vi "contains.vi"(0 "reference":refnum<class "PackageNode.lvclass">, 1 "point2D":T1 {"y" format="%.2f"; "x" format="%.2f"}, 2 "AdditionalMargin":i32, 5 "error in (no error)":errorcluster) -> (14 "reference out":refnum<class "PackageNode.lvclass">, 15 "contains":bool, 19 "error out":errorcluster)   [LabVIEW 2014, in "PackageNode.lvclass"]
doc: "contains"
uses:
  <resource>/Framework/Providers/Open_GDS/UML/PackageNode_class/PackageNode.lvclass
  <resource>/Framework/Providers/Open_GDS/UML/General/Point/Point Point2D.ctl
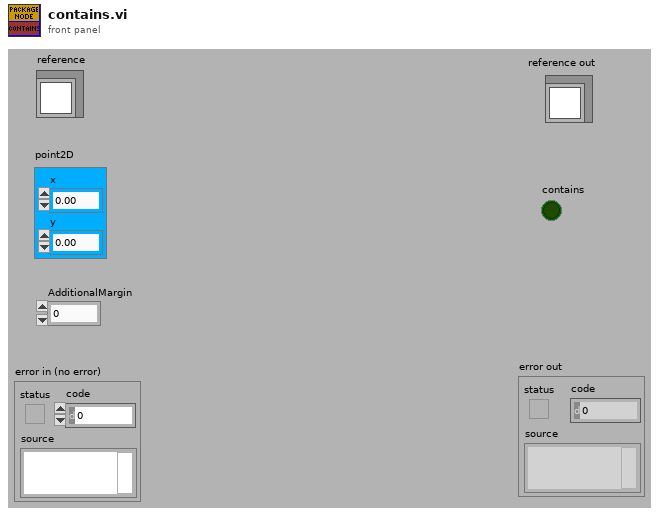
[diagram p1: front panel]
types:
  T1 = typedef "Point Point2D.ctl" = cluster{"x":dbl, "y":dbl}
  T2 = typedef "PackageNode.lvclass/ObjectAttributes.ctl" = cluster{"Base class":T3, "name":string, "contents":refnum<class "MultiLineString.lvclass">, "DEFAULT_TOP_WIDTH":i32, "DEFAULT_TOP_HEIGHT":i32, "DEFAULT_WIDTH":i32, "DEFAULT_HEIGHT":i32, "NAME_GAP":i32, "XGAP":i32, "YGAP":i32, "Collapsed":bool, "Note color":u32, "Justification":u16}
  T3 = typedef "RectangularNode.lvclass/ObjectAttributes.ctl" = cluster{"Base class":T4, "bounds":T5}
  T4 = typedef "AbstractNode.lvclass/ObjectAttributes.ctl" = cluster{"parent":refnum<class "AbstractNode.lvclass">, "children":refnum<class "AbstractNode.lvclass">[], "Hidden":bool}
  T5 = typedef "Rectangle Rectangle2D.ctl" = cluster{"x":dbl, "y":dbl, "width":dbl, "height":dbl}
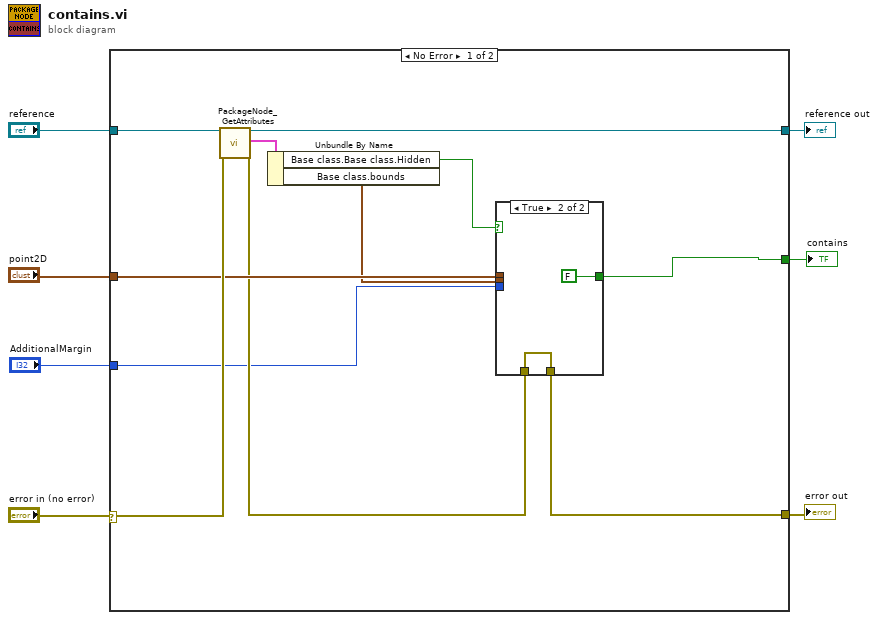
[diagram p0: block diagram]
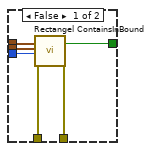
[diagram p2: hidden frame]
diagram:
  n1 = case shown="No Error" "error in (no error)" {
    selector: "error in (no error)" -> [w15 w27]
    tunnel: "reference" -> [w18 w28]
    tunnel: [w17 w27] -> w6
    tunnel: [w16 w28] -> w5
    tunnel: "point2D" -> [w14 _]
    tunnel: [w13 _] -> w2
    tunnel: "AdditionalMargin" -> [w9 _]
    frame No Error {
      n2 = call <resource>:"PackageNode_GetAttributes.vi"("reference in"=w18, "error in (no error)"=w15) -> ("reference out"=w16:refnum<class "PackageNode.lvclass">, "Attributes"=w12:T2, "error out"=w10:errorcluster)  [unwired: 14 in, 1 out]
      n3 = Unbundle By Name(w12) -> ("Base class.Base class.Hidden"=w8:bool, "Base class.bounds"=w11:T5)
      n4 = case shown="True" w8 {
        tunnel: [w24 w26] -> w17
        tunnel: w14 -> [w23 _]
        tunnel: [w22 FALSE ("contains")] -> w13
        tunnel: w11 -> [w21 _]
        tunnel: w10 -> [w20 w26]
        tunnel: w9 -> [w19 _]
        frame False {
          n5 = call <resource>:"Rectangel ContainsInBound.vi"("point2D"=w23, "bounds"=w21, "AdditionalMargin"=w19, "error in (no error)"=w20) -> ("contains"=w22:bool, "error out"=w24:errorcluster)  [unwired: 14 out]
        }
        frame True {
        }
      }
    }
    frame Error {
    }
  }
  "reference out" <- w5
  "error out" <- w6
  "contains" <- w2
